vi "FindExp.vi"(10 "extension name":string, 11 "lang_font.exp":string) -> (3 "spreadsheet string":string)   [LabVIEW 2019]
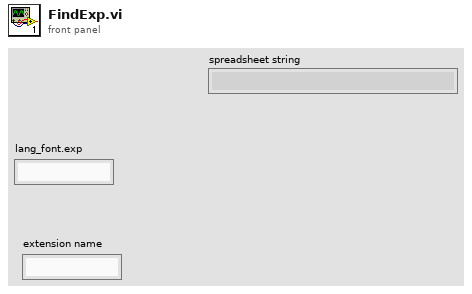
[diagram p1: front panel]
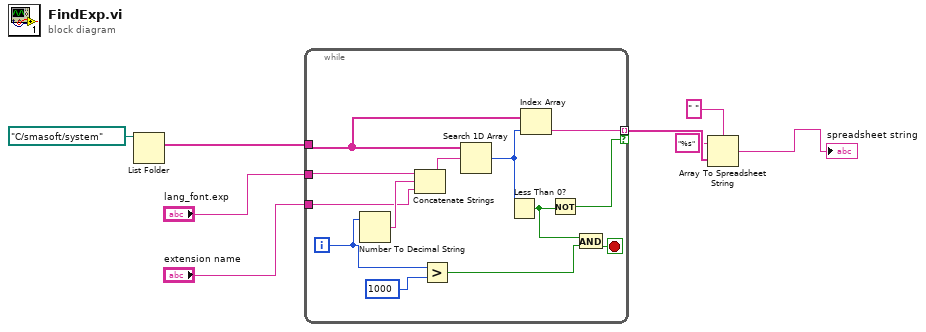
[diagram p0: block diagram]
diagram:
  n1 = List Folder(path=path "C:/smasoft/system") -> (filenames=w7:string[])  [unwired: 3 in, 3 out]
  n2 = while {
    tunnel: w7 -> [w18]
    tunnel: "lang_font.exp" -> [w20]
    tunnel: "extension name" -> [w9]
    tunnel: [w17] -> w4 mode=indexing if=w12
    i -> [w15]
    stop <- w13 stop-if-true
    n3 = Number To Decimal String(number=w15) -> (decimal integer string=w19:string)  [unwired: 1 in]
    n4 = Concatenate Strings(w20, w19, w9) -> (w21:string)
    n5 = Greater?(x=w15, y=1000) -> (0:w11:bool)
    n6 = Search 1D Array(1D array=w18, element=w21) -> (index of element=w16:i32)  [unwired: 1 in]
    n7 = Less Than 0?(x=w16) -> (x < 0?=w10:bool)
    n8 = Index Array(array=w18, index=w16) -> (element=w17:string)
    n9 = Not(x=w10) -> (.not. x?=w12:bool)
    n10 = And(x=w10, y=w11) -> (x .and. y?=w13:bool)
  }
  n11 = Array To Spreadsheet String(delimiter (Tab)=" ", array=w4, 3:"%s" ("format string")) -> (spreadsheet string=→"spreadsheet string":string)
